vi "Receive ILC Inputs.vi"(8 "error in (no error)":errorcluster, 11 "Model in":refnum<class "Model.lvclass">) -> (0 "error out":errorcluster, 3 "Model out":refnum<class "Model.lvclass">)   [LabVIEW 2016, in "Model.lvclass"]
uses:
  Model.lvclass
  Model.lvclass/Model.ctl
  common_rt_modbus/DynamicFrameParser/DynamicFrameParser.lvclass
  Modbus/DesktopModbus/DesktopModbus.lvclass
  common_rt_hpilc/HPILC/HPILC.lvclass
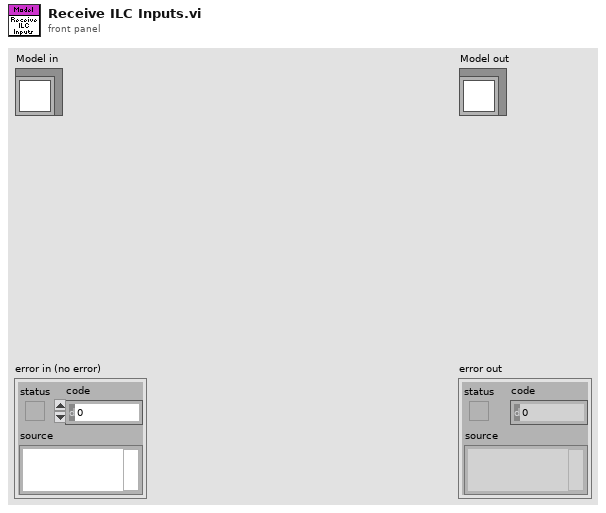
[diagram p1: front panel]
types:
  T1 = typedef "RTModbus.lvlib/RxFrame.ctl" = cluster{"Data":u8[], "Timestamp":u64}
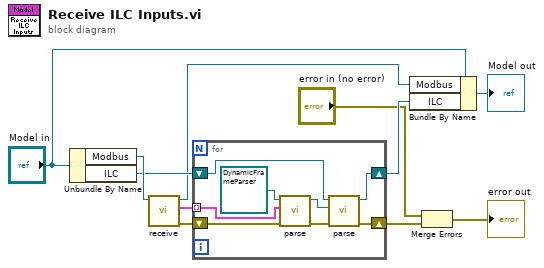
[diagram p0: block diagram]
diagram:
  n1 = Unbundle By Name("Model in") -> ("Modbus"=w11:refnum<class "DesktopModbus.lvclass">, "ILC"=w9:refnum<class "HPILC.lvclass">)
  n2 = call-dynamic "receive.vi"("DesktopModbus in"=w11) -> ("error out"=w5:errorcluster, "Data"=w10:T1[], "DesktopModbus out"=w7:refnum<class "DesktopModbus.lvclass">)  [unwired: 8 in]
  n3 = for {
    tunnel: w10 -> [w18] mode=indexing
    shift-right: [w15] -> w6
    shift-left: w9 -> [w16]
    shift-right: [w12] -> w2
    shift-left: w5 -> [w17]
    n4 = call "parse.vi"("error in (no error)"=w17, "RxFrame"=w18, "FrameParser in"=refnum<class "DynamicFrameParser.lvclass"> refnum ("RTModbus.lvlib:DynamicFrameParser.lvclass")) -> ("error out"=w13:errorcluster, "FrameParser out"=w14:refnum<class "DynamicFrameParser.lvclass">)  [unwired: 7 in]
    n5 = call-dynamic "parse.vi"("error in (no error)"=w13, "DynamicFrameParser"=w14, "HPILC in"=w16) -> ("error out"=w12:errorcluster, "HPILC out"=w15:refnum<class "HPILC.lvclass">)  [unwired: 6 in, 1 out]
  }
  n6 = Bundle By Name(cluster="Model in", "Modbus"=w7, "ILC"=w6) -> (→"Model out":refnum<class "Model.lvclass">)
  n7 = Merge Errors("error in (no error)", w2) -> (→"error out":errorcluster)
